vi "ClkRegTest.vi"(0 "COMPORT":refnum<visa-resource-name>="COM5", 5 "PyScript(path)":path=path "C:/Labview/Projects/WAM_CLK_TEST/support_files/VerifySiTime.py", 9 "WamGood(path)":path=path "C:/Labview/Projects/WAM_CLK_TEST/support_files/ext_wamGood.txt", 11 "error in":errorcluster) -> (2 "P/F(bool)":bool, 3 "P/F(str)":string, 4 "result string":string, 15 "error out":errorcluster)   [LabVIEW 2018]
panel:
  out "Message":string
  out "All Success":bool
  out "comp string":string
  out "ok?(t)":bool
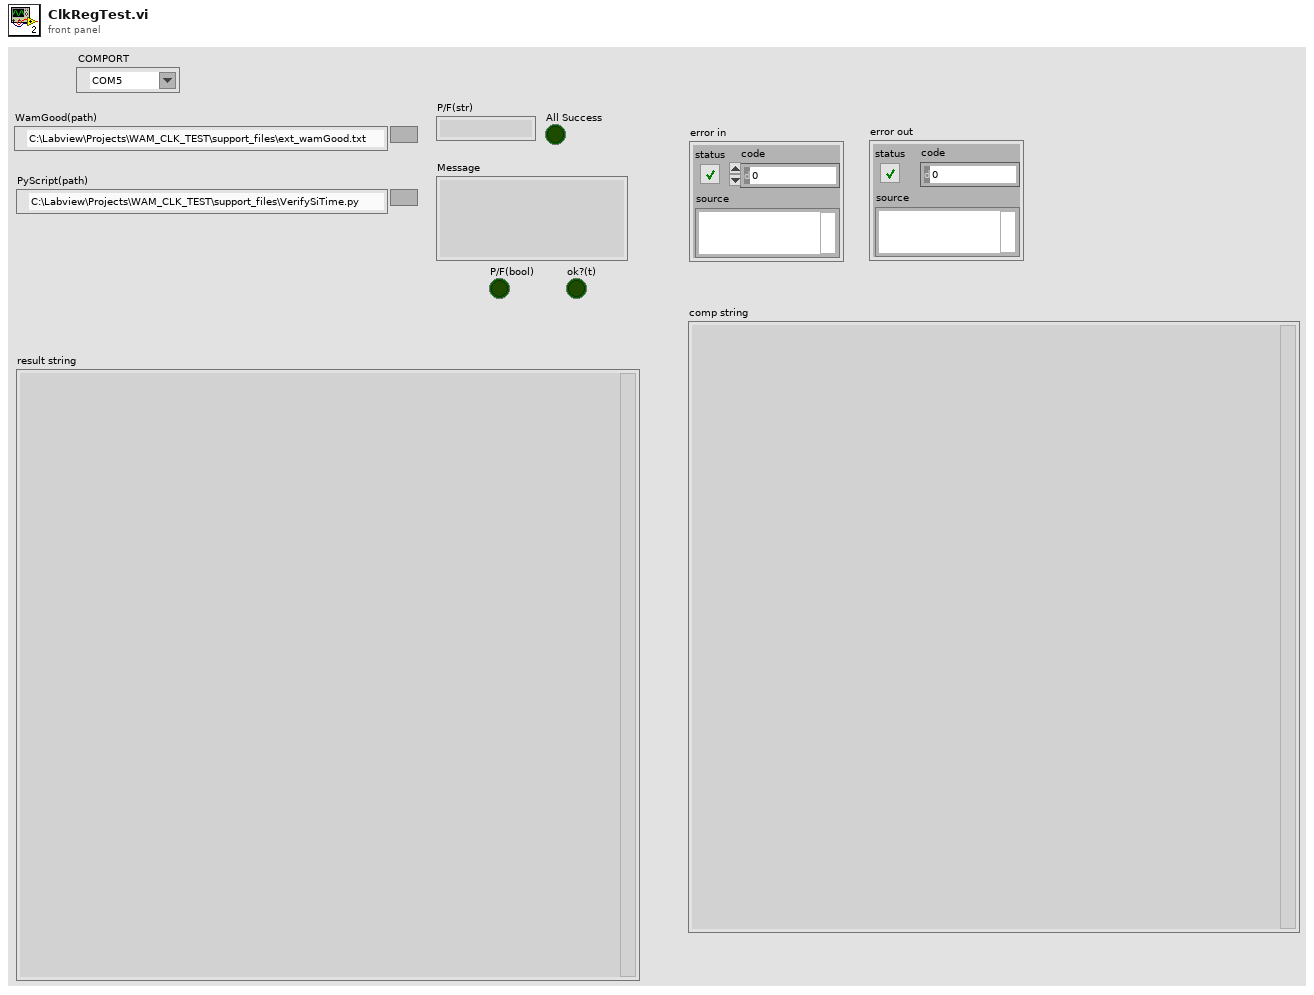
[diagram p1: front panel]
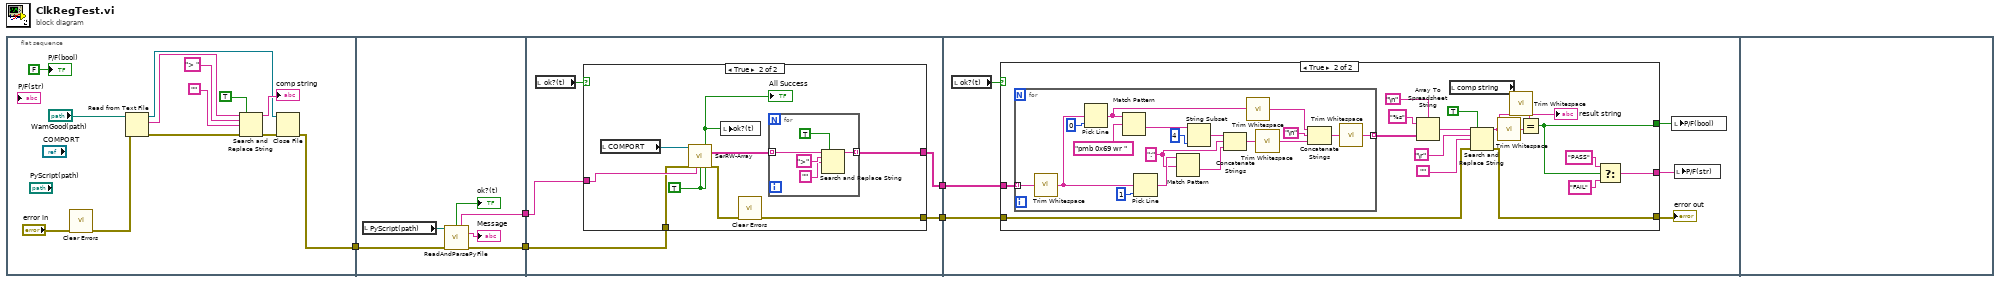
[diagram p0: block diagram]
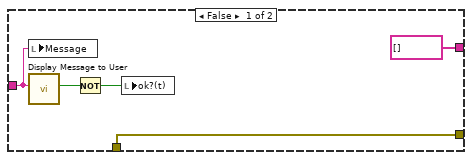
[diagram p2: hidden frame]
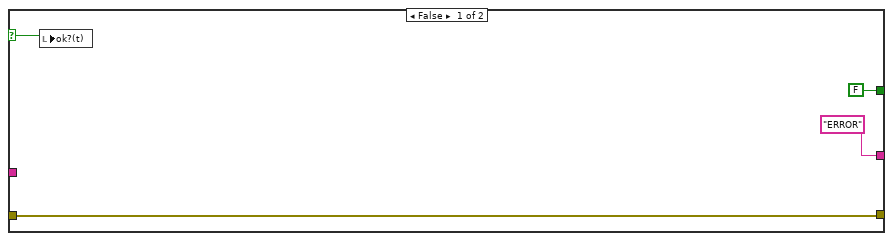
[diagram p3: hidden frame]
diagram:
  n1 = flat-sequence {
    tunnel: [w6] -> w3
    tunnel: [w23] -> w5
    tunnel: w3 -> [w20]
    tunnel: [w19] -> w2
    tunnel: w5 -> [w29]
    tunnel: [w28] -> w4
    tunnel: w2 -> [w26]
    tunnel: [w25] -> w1
    tunnel: w4 -> [w54]
    tunnel: w1 -> [w50]
    frame #0 {
      n2 = call <vilib>:"Clear Errors.vi"("error in (no error)"="error in") -> ("error out"=w7:errorcluster)  [unwired: 5 in, 1 out]
      n3 = Read from Text File(file (use dialog)="WamGood(path)", error in=w7) -> (refnum out=w12:refnum<file>, text=w17:string, error out=w10:errorcluster)  [unwired: 2 in, 1 out]
      n4 = Search and Replace String(replace all?=TRUE ("replace all? (F)"), input string=w17, search string="> ", replace string="", error in=w10) -> (result string=→"comp string":string, error out=w11:errorcluster)  [unwired: 3 in, 2 out]
      n5 = Close File(refnum=w12, error in=w11) -> (error out=w6:errorcluster)  [unwired: 1 out]
      "P/F(bool)" <- FALSE ("P/F(bool)")
    }
    frame #1 {
      n6 = local read "PyScript(path)"() -> (w22:path)
      n7 = call "ReadAndParsePyFile.vi"("file path (dialog if empty)"=w22, "error in (no error)"=w20) -> ("ok?(t)"=→"ok?(t)":bool, "regs"=w23:string, "Message"=→"Message":string, "error out"=w19:errorcluster)  [unwired: 10 in]
    }
    frame #2 {
      n8 = local read "ok?(t)"() -> (w27:bool)
      n9 = case shown="True" w27 {
        tunnel: w29 -> [w31 w43]
        tunnel: [string[] [] w40] -> w28
        tunnel: w26 -> [w30 w37]
        tunnel: [w30 w35] -> w25
        frame False {
          n10 = local write "Message"(w31) -> ()
          n11 = call "Display Message to User"("Message"=w31) -> ("OK"=w34:bool)  [unwired: 9 in, 1 out]
          n12 = Not(x=w34) -> (.not. x?=w33:bool)
          n13 = local write "ok?(t)"(w33) -> ()
        }
        frame True {
          w42 = TRUE ("Open Serial")
          n14 = local read "COMPORT"() -> (w39:refnum<visa-resource-name>)
          n15 = call "SerRW-Array.vi"("COMPORT"=w39, "error in (no error)"=w37, "Command ( ; seperation)"=w43, "Open Serial"=w42, "Close Serial"=w42) -> ("All Success"=w38:bool, "Array"=w41:string[], "error out"=w36:errorcluster)  [unwired: 4 in, 4 out]
          "All Success" <- w38
          n16 = local write "ok?(t)"(w38) -> ()
          n17 = call <vilib>:"Clear Errors.vi"("error in (no error)"=w36) -> ("error out"=w35:errorcluster)  [unwired: 5 in, 1 out]
          n18 = for {
            tunnel: w41 -> [w45] mode=indexing
            tunnel: [w44] -> w40 mode=indexing
            n19 = Search and Replace String(replace all?=TRUE ("replace all? (F)"), input string=w45, search string=">", replace string="") -> (result string=w44:string)  [unwired: 4 in, 3 out]
          }
        }
      }
    }
    frame #3 {
      n20 = local read "ok?(t)"() -> (w51:bool)
      n21 = case shown="True" w51 {
        selector: w51 -> [w56 _]
        tunnel: w54 -> [_ w75]
        tunnel: [FALSE w72] -> w53
        tunnel: ["ERROR" w71] -> w52
        tunnel: w50 -> [w55 w62]
        tunnel: [w55 w61] -> w49
        frame False {
          n22 = local write "ok?(t)"(w56) -> ()
        }
        frame True {
          n23 = for {
            tunnel: [w80] -> w68 mode=indexing
            tunnel: w75 -> [w79] mode=indexing
            w87 = ":" ("regular expression")
            n24 = call <vilib>:"Trim Whitespace.vi"("string"=w79) -> ("trimmed string"=w81:string)  [unwired: 1 in]
            n25 = Pick Line(multi-line string=w81, line index=0) -> (output string=w94:string)  [unwired: 1 in]
            n26 = Match Pattern(string=w94, regular expression="pmb 0x69 wr ") -> (after substring=w89:string)  [unwired: 1 in, 3 out]
            n27 = Pick Line(multi-line string=w81, line index=1) -> (output string=w90:string)  [unwired: 1 in]
            n28 = Match Pattern(string=w90, regular expression=w87) -> (after substring=w91:string)  [unwired: 1 in, 3 out]
            n29 = String Subset(string=w89, length (rest)=4 ("length (rest)")) -> (substring=w92:string)  [unwired: 1 in]
            n30 = Concatenate Strings(w92, w87, w91) -> (w93:string)
            n31 = call <vilib>:"Trim Whitespace.vi"("string"=w94) -> ("trimmed string"=w78:string)  [unwired: 1 in]
            n32 = call <vilib>:"Trim Whitespace.vi"("string"=w93) -> ("trimmed string"=w77:string)  [unwired: 1 in]
            n33 = Concatenate Strings(w78, "\n", w77) -> (w82:string)
            n34 = call <vilib>:"Trim Whitespace.vi"("string"=w82) -> ("trimmed string"=w80:string)  [unwired: 1 in]
          }
          n35 = Array To Spreadsheet String(delimiter (Tab)="\n", array=w68, 3:"%s" ("format string")) -> (spreadsheet string=w70:string)
          n36 = local read "comp string"() -> (w69:string)
          n37 = Search and Replace String(replace all?=TRUE ("replace all? (F)"), input string=w70, search string="\r", replace string="", error in=w62) -> (result string=w76:string, error out=w61:errorcluster)  [unwired: 3 in, 2 out]
          "result string" <- w76
          n38 = call <vilib>:"Trim Whitespace.vi"("string"=w76) -> ("trimmed string"=w60:string)  [unwired: 1 in]
          n39 = call <vilib>:"Trim Whitespace.vi"("string"=w69) -> ("trimmed string"=w59:string)  [unwired: 1 in]
          n40 = Equal?(x=w59, y=w60) -> (x = y?=w72:bool)
          n41 = Select(t="PASS", s=w72, f="FAIL") -> (s? t:f=w71:string)
        }
      }
      "error out" <- w49
      n42 = local write "P/F(bool)"(w53) -> ()
      n43 = local write "P/F(str)"(w52) -> ()
    }
    frame #4 {
    }
  }
